vi "ProdaNG.ProcessResult.Get.vi"(8 "error in (no error)":errorcluster, 9 "processId":i32, 10 "productId":string, 11 "dbHandle":i32) -> (0 "error out":errorcluster, 1 "Found":bool, 2 "ProcessResult":T1, 3 "dbHandle out":i32)   [LabVIEW 2016]
doc: "This function returns a ProcessResult structure for a product in a process. \nParameter:\nhandle is an Integer, which is returned by the function Login() at the creation of a new connection.\nproductId is the Id of the associated product.\nprocessId is the Id of the associated process.\nprocessResult is a pointer on a processResult structure, which is filled if the returncode is 0. The structure must be defined in the calling program.\nReturncodes:\n0 No error\n< 0 ORACLE Error code\n6 (ERROR_INVALID_HANDLE) in case of an invalid handle\n1403 Record does not exist"
uses:
  Controls/ProdaNG.ProcessResult.ctl
  Controls/ProdaNG.ProcessResultSize.ctl
  prodllNG.dll
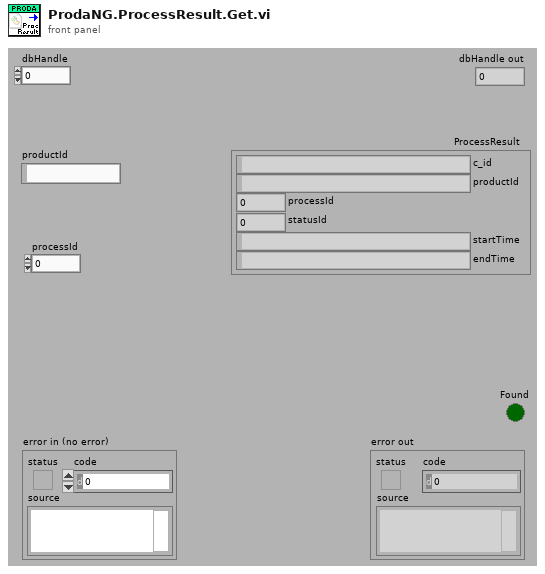
[diagram p1: front panel]
types:
  T1 = typedef "ProdaNG.ProcessResult.ctl" = cluster{"c_id":string, "productId":string, "processId":i32, "statusId":i32, "startTime":string, "endTime":string}
  T2 = typedef "ProdaNG.ProcessResultSize.ctl" = cluster{"c_id":i32, "productId":i32, "processId":i32, "statusId":i32, "startTime":i32, "endTime":i32}
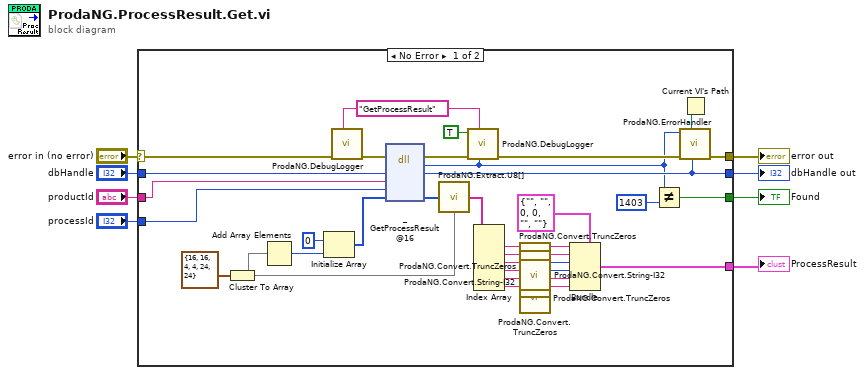
[diagram p0: block diagram]
diagram:
  n1 = case shown="No Error" "error in (no error)" {
    selector: "error in (no error)" -> [w37 w46]
    tunnel: [w42 w46] -> w7
    tunnel: "dbHandle" -> [w44 w45]
    tunnel: [w40 w45] -> w5
    tunnel: "productId" -> [w43 _]
    tunnel: "processId" -> [w33 _]
    tunnel: [w24 _] -> w4
    tunnel: [w22 _] -> w1
    frame No Error {
      w39 = "GetProcessResult" ("cmd")
      n2 = Cluster To Array(cluster=T2 {"c_id"=16, "productId"=16, "processId"=4, "statusId"=4, "startTime"=24, "endTime"=24} ("ProcessResultSize")) -> (array=w28:i32[])
      n3 = Add Array Elements(numeric array=w28) -> (sum=w31:i32)
      n4 = Initialize Array(u8 0 ("element"), w31) -> (w27:u8[])
      n5 = call "ProdaNG.DebugLogger.vi"("cmd"=w39, "error in (no error)"=w37) -> ("error out"=w36:errorcluster)  [unwired: 9 in]
      n6 = dll-call lib="D:/svn/LineTraceSystem/SOFTWARE/sources/Database/ProdaNG/prodllNG.dll" fn="_GetProcessResult@16" ("ProDLL wrapper.dll:ProDLL_wrapper_GetWabcoParts_GetData")(error in=w36, "dbHandle"=w44, "productId"=w43, "processId"=w33, "processResult"=w27) -> (error out=w35:errorcluster, "return type"=w25:i32, "dbHandle"=w40:i32, "processResult"=w26:u8[])  [unwired: 4 in, 1 out]
      n7 = call "ProdaNG.Extract.U8[].vi"("unsigned byte array"=w26, "Sizes"=w28) -> ("Elements"=w30:string[])
      n8 = call "ProdaNG.DebugLogger.vi"("return type"=w25, "cmd"=w39, "error in (no error)"=w35, "done? (F)"=TRUE) -> ("error out"=w34:errorcluster)  [unwired: 7 in]
      n9 = Index Array(array=w30) -> (element #1=w11:string, element #2=w10:string, element #3=w21:string, element #4=w18:string, element #5=w15:string, element #6=w17:string)  [unwired: 6 in]
      n10 = call "ProdaNG.Convert.TruncZeros.vi"("string with \\0s"=w11) -> ("LV string"=w13:string)  [unwired: 10 in]
      n11 = call "ProdaNG.Convert.TruncZeros.vi"("string with \\0s"=w10) -> ("LV string"=w12:string)  [unwired: 10 in]
      n12 = call "ProdaNG.Convert.String-I32.vi"("unsigned byte string"=w21) -> ("32bit integer"=w20:i32)  [unwired: 10 in]
      n13 = call "ProdaNG.Convert.String-I32.vi"("unsigned byte string"=w18) -> ("32bit integer"=w19:i32)  [unwired: 10 in]
      n14 = call "ProdaNG.Convert.TruncZeros.vi"("string with \\0s"=w15) -> ("LV string"=w14:string)  [unwired: 10 in]
      n15 = call "ProdaNG.Convert.TruncZeros.vi"("string with \\0s"=w17) -> ("LV string"=w16:string)  [unwired: 10 in]
      n16 = Bundle(cluster=T1 {"c_id"="", "productId"="", "processId"=0, "statusId"=0, "startTime"="", "endTime"=""} ("ProcessResult"), "c_id"=w13, "productId"=w12, "processId"=w20, "statusId"=w19, "startTime"=w14, "endTime"=w16) -> (w22:T1)
      n17 = Not Equal?(x=w25, y=1403) -> (x != y?=w24:bool)
      n18 = Current VI's Path() -> (path=w41:path)
      n19 = call "ProdaNG.ErrorHandler.vi"("dbHandleIn"=w40, "Path"=w41, "error in"=w34, "output_parameter"=w25) -> ("error out"=w42:errorcluster)  [unwired: 7 in]
    }
    frame Error {
    }
  }
  "error out" <- w7
  "dbHandle out" <- w5
  "Found" <- w4
  "ProcessResult" <- w1
